vi "Global 1.vi"() -> ()   [LabVIEW 2016]
panel:
  in  "tmp 2":i32
  in  "Исходное сообщение":string
  in  "Зашифрованный ключ_р":i32[][](array[numeric])
  in  "tmp":i32
  in  "Count_col":i32
  in  "Вх. масс. алф.":string[][](array[string])
  in  "Зашифрованный вектор":i32[](array[numeric])
  in  "Зашифрованное сообщение":i32[](array[numeric])
  in  "Расшифрованный вектор":i32[](array[numeric])
  in  "Матрица ключа":i32[][](array[numeric])
  in  "Вх. алф. расшифр.":string
  in  "Длина  вх. алфавита":i32
  in  "Вектор входного слова":i32[](array[numeric])
  in  "Входной алфавит":string
  in  "index":i32[](array[numeric])
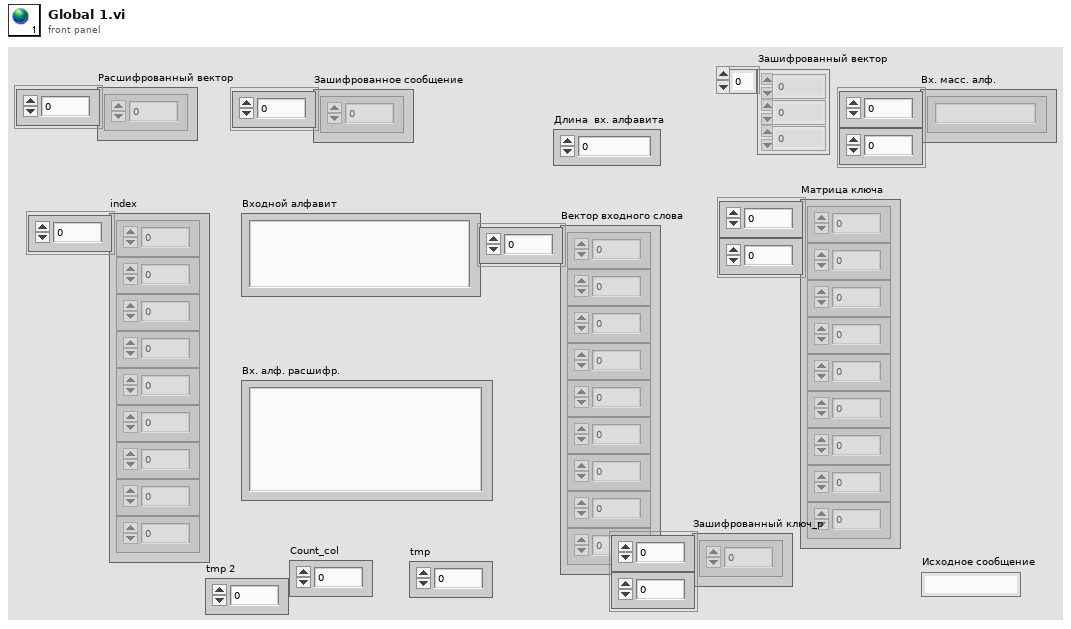
[diagram p1: front panel]
diagram:
